vi "DockGUI.vi"(8 "ErrorIn":errorcluster, 9 "SubPanelName":string, 10 "ObjectName":string, 11 "ReferenceIn":refnum<class "MasterGUI.lvclass">) -> (0 "ErrorOut":errorcluster, 3 "ReferenceIn":refnum<class "MasterGUI.lvclass">)   [LabVIEW 2021, in "MasterGUI.lvclass"]
uses:
  MasterGUI.lvclass
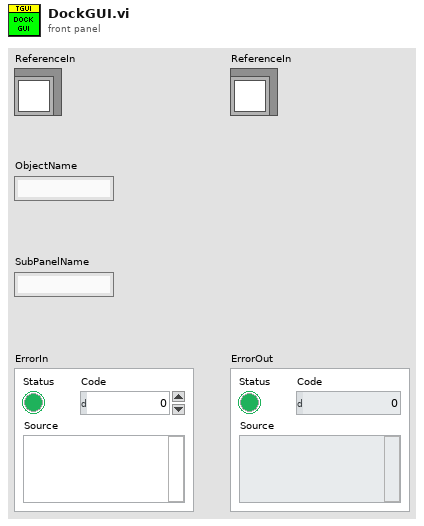
[diagram p1: front panel]
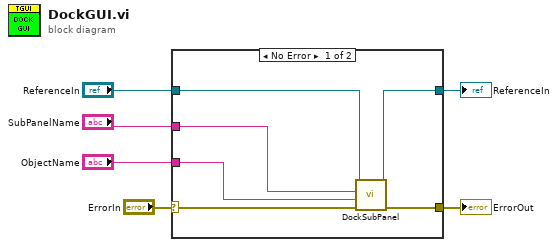
[diagram p0: block diagram]
diagram:
  n1 = case shown="No Error" "ErrorIn" {
    selector: "ErrorIn" -> [w11 w14]
    tunnel: [w12 w14] -> w5
    tunnel: [w9 w13] -> w3
    tunnel: "ReferenceIn" -> [w10 w13]
    tunnel: "SubPanelName" -> [w8 _]
    tunnel: "ObjectName" -> [w7 _]
    frame No Error {
      n2 = call-dynamic "DockSubPanel.vi"("ErrorIn"=w11, "ObjectLabel"=w7, "PanelLabel"=w8, "ReferenceIn"=w10) -> ("ErrorOut"=w12:errorcluster, "ReferenceIn"=w9:refnum<class "MasterGUI.lvclass">)  [unwired: 6 in]
    }
    frame Error {
    }
  }
  "ErrorOut" <- w5
  "ReferenceIn" <- w3
